vi "Coral Command.vi"(3 "Synchronization":enum16{"Start", "Wait"}(ring), 4 "Description":string, 5 "Command Info In":T1, 6 "Positional Array":dbl[](array[numeric]), 7 "Setpoint State":T4=enum."L2", 8 "Confirm or Negate":bool, 9 "Coral States":T5, 10 "Operation":T6) -> (0 "Command Info Out":T1)   [LabVIEW 2023]
uses:
  Implementation/Coral Operations.ctl
  Support Code/Teleop Util/Coral States.ctl
  <vilib>/Rock Robotics/WPI/Framework/Command Status Info.ctl
  <vilib>/Rock Robotics/WPI/Framework/Completion Status.ctl
  <vilib>/Rock Robotics/WPI/Framework/Completion Notifier.ctl
  Support Code/Teleop Util/Scoring Levels.ctl
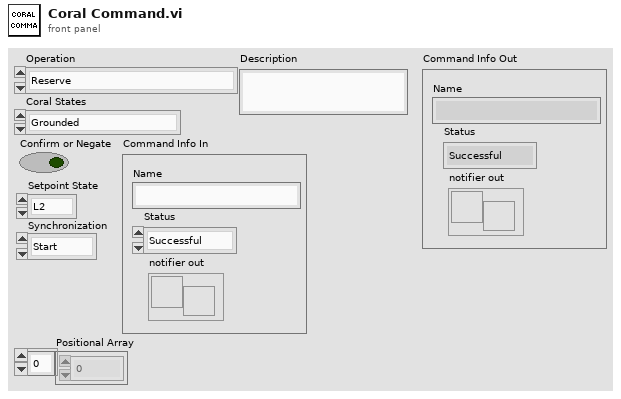
[diagram p1: front panel]
types:
  T1 = typedef "Command Status Info.ctl" = cluster{"Name":string, "Status":T2, "notifier out":T3}
  T2 = typedef "Completion Status.ctl" = enum16{"Successful", "Aborted", "Incomplete"}
  T3 = typedef "Completion Notifier.ctl" = refnum<notifier>
  T4 = typedef "Scoring Levels.ctl" = enum16{"Trough", "L2", "L3", "L4", "Default"}
  T5 = typedef "Coral States.ctl" = enum16{"Grounded", "Coral Intake", "Scoring Sequence", "Hold Position", "Score", "Manual Override", "Climb Safety Mode"}
  T6 = typedef "Coral Operations.ctl" = enum16{"Reserve", "Read Current", "Immediate", "Calibrate"}
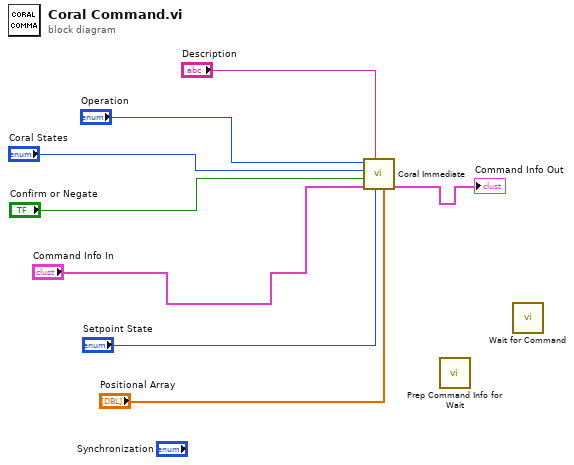
[diagram p0: block diagram]
diagram:
  n1 = call "Coral Immediate.vi"("Positional Array"="Positional Array", "Setpoint State"="Setpoint State", "Description"="Description", "Command Info In"="Command Info In", "Confirm or Negate"="Confirm or Negate", "Coral States"="Coral States", "Operation"="Operation") -> ("Command Info Out"=→"Command Info Out":T1)  [unwired: 4 in]
  n2 = call <vilib>:"Prep Command Info for Wait.vi"() -> ()  [unwired: 10 in, 2 out]
  n3 = call <vilib>:"Wait for Command.vi"() -> ()  [unwired: 11 in, 1 out]
